vi "HEWH Emerson Data.vi"(7 "Status":T2, 8 "error in (no error)":errorcluster, 10 "Emerson Flow Meter Data Input":T1, 11 "name (unnamed)":string) -> (0 "error out":errorcluster, 3 "Emerson Flow Meter Data Output":T1)   [LabVIEW 2019]
uses:
  Utility/Type Definitions/UTILITY Notifier.ctl
  Drivers/Emerson 5700 Transmitter/Type Definitions/Emerson 5700 Data.ctl
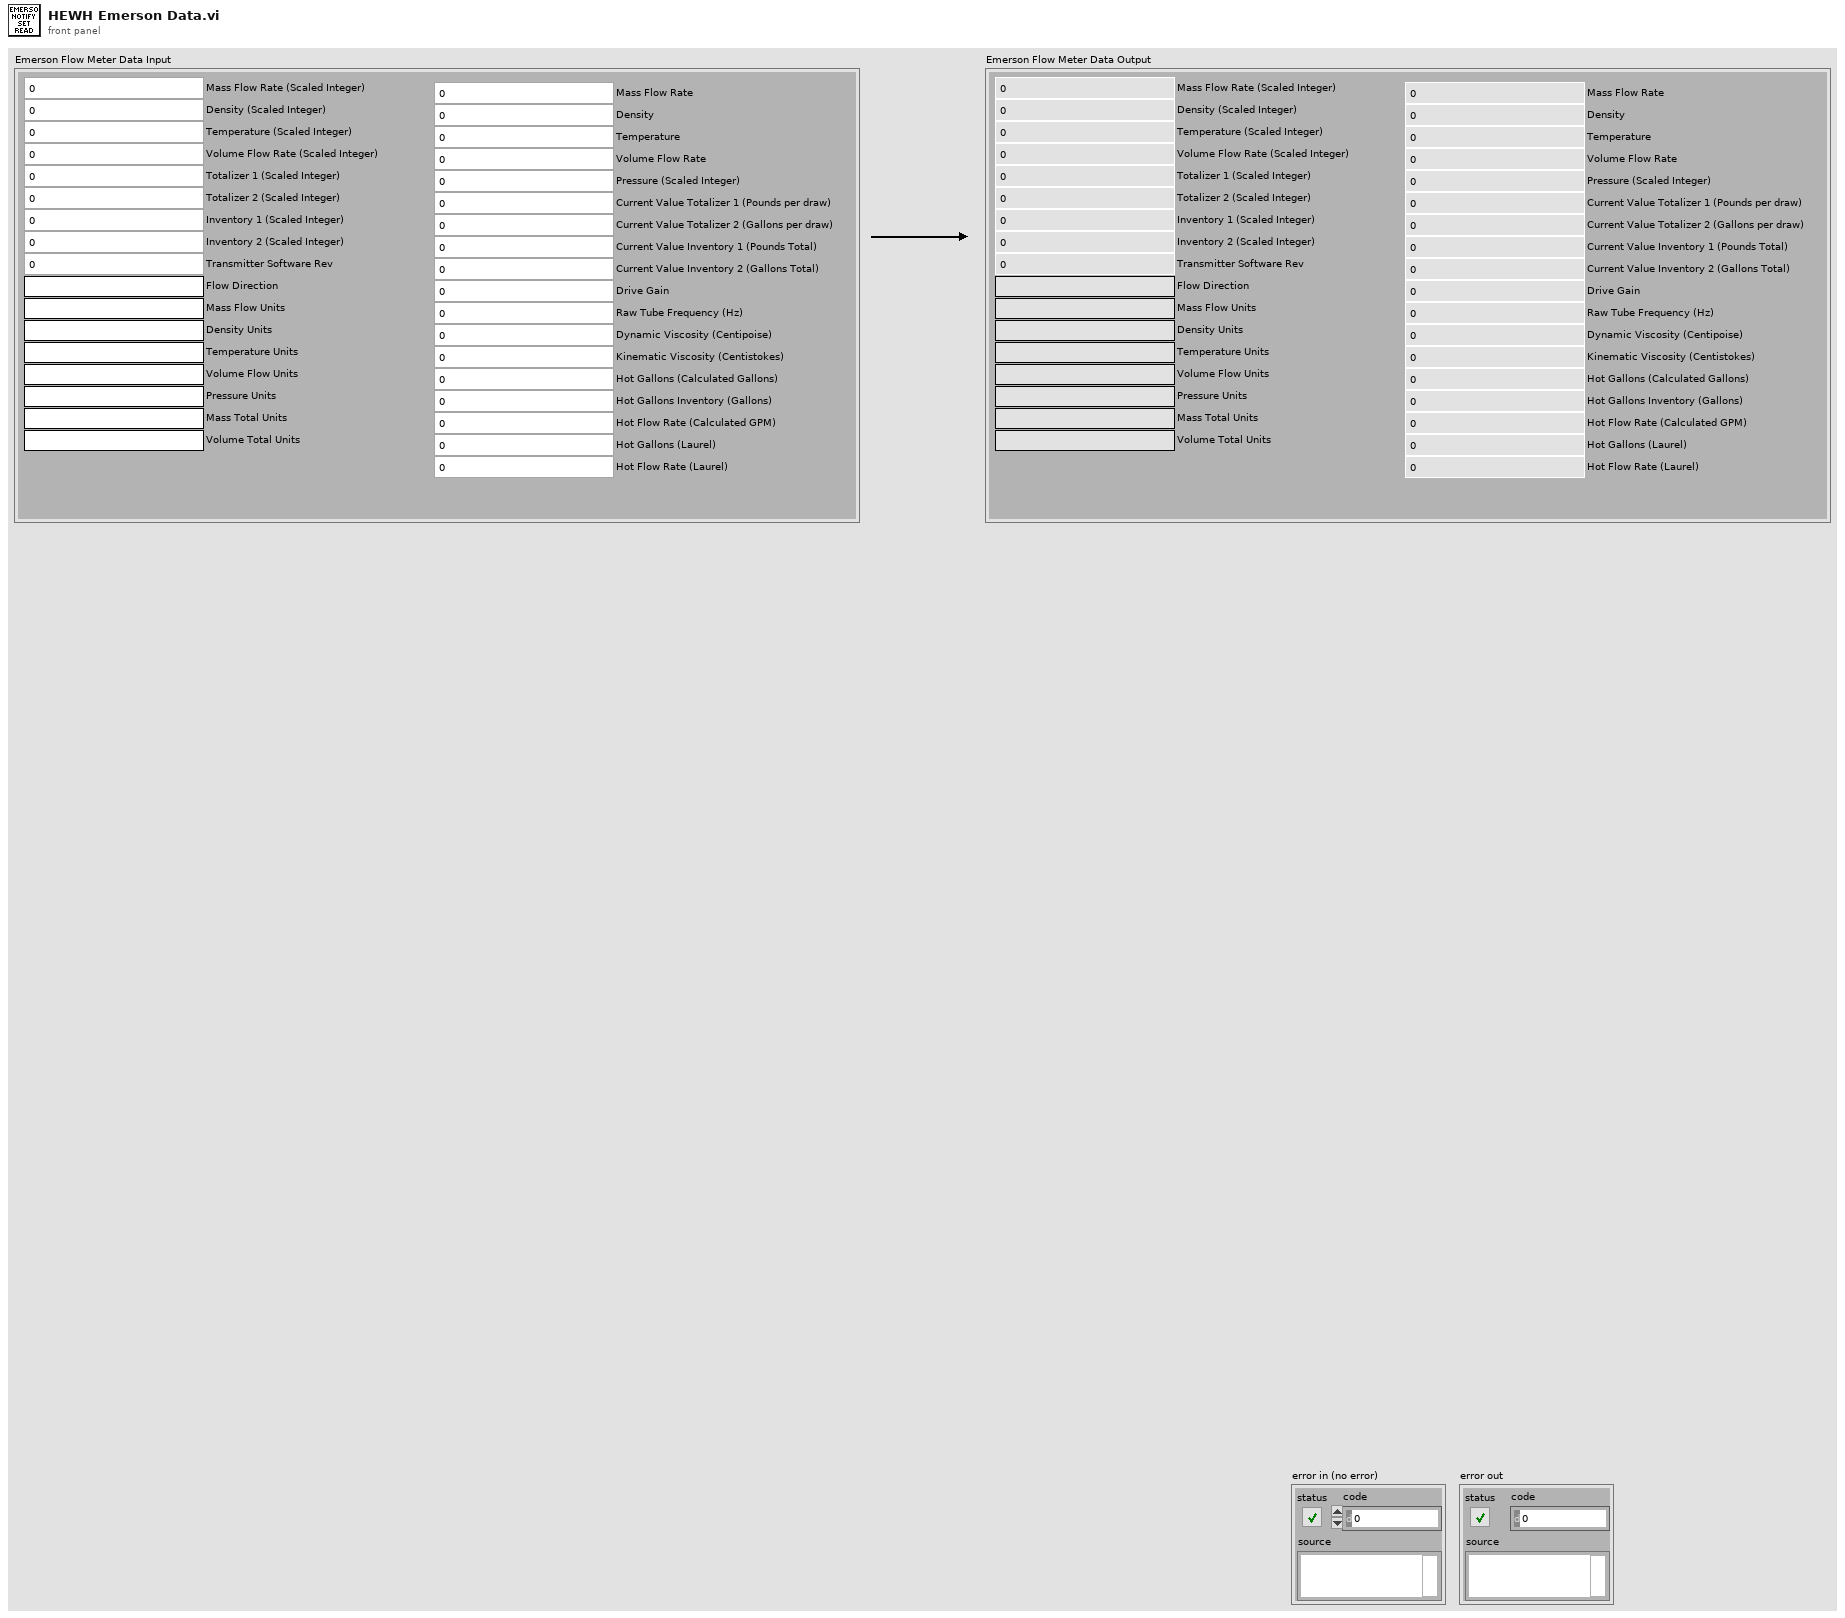
[diagram p1: front panel]
types:
  T1 = typedef "Emerson 5700 Data.ctl" = cluster{"Mass Flow Rate (Scaled Integer)":u16, "Density (Scaled Integer)":u16, "Temperature (Scaled Integer)":u16, "Volume Flow Rate (Scaled Integer)":u16, "Totalizer 1 (Scaled Integer)":u16, "Totalizer 2 (Scaled Integer)":u16, "Transmitter Software Rev":u16, "Flow Direction":string, "Mass Flow Units":string, "Density Units":string, "Temperature Units":string, "Volume Flow Units":string, "Pressure Units":string, "Mass Total Units":string, "Volume Total Units":string, "Inventory 1 (Scaled Integer)":u16, "Inventory 2 (Scaled Integer)":u16, "Mass Flow Rate":dbl, "Density":dbl, "Temperature":dbl, "Volume Flow Rate":dbl, "Pressure (Scaled Integer)":u16, "Current Value Totalizer 1 (Pounds per draw)":dbl, "Current Value Totalizer 2 (Gallons per draw)":dbl, "Current Value Inventory 1 (Pounds Total)":dbl, "Current Value Inventory 2 (Gallons Total)":dbl, "Drive Gain":dbl, "Raw Tube Frequency (Hz)":dbl, "Dynamic Viscosity (Centipoise)":dbl, "Kinematic Viscosity (Centistokes)":dbl, "Hot Gallons (Calculated Gallons)":dbl, "Hot Flow Rate (Calculated GPM)":dbl, "Hot Gallons Inventory (Gallons)":dbl, "Hot Flow Rate (Laurel)":dbl, "Hot Gallons (Laurel)":dbl}
  T2 = typedef "UTILITY Notifier.ctl" = enum16{"Set", "Read", "Release Ref"}
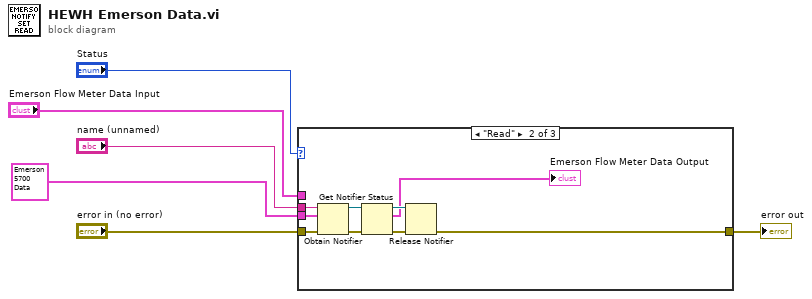
[diagram p0: block diagram]
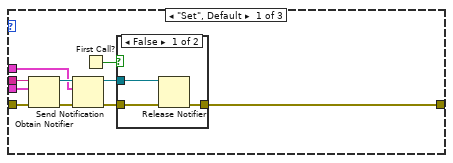
[diagram p2: hidden frame]
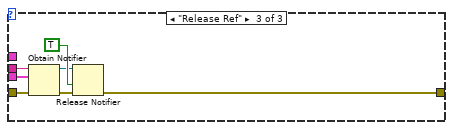
[diagram p4: hidden frame]
diagram:
  n1 = case shown="\"Read\"" "Status" {
    tunnel: [w7 w23 w32] -> w6
    tunnel: "error in (no error)" -> [w14 w27 w33]
    tunnel: "name (unnamed)" -> [w13 w26 w31]
    tunnel: T1 {"Mass Flow Rate (Scaled Integer)"=0, "Density (Scaled Integer)"=0, "Temperature (Scaled Integer)"=0, "Volume Flow Rate (Scaled Integer)"=0, "Totalizer 1 (Scaled Integer)"=0, "Totalizer 2 (Scaled Integer)"=0, "Transmitter Software Rev"=0, "Flow Direction"="", "Mass Flow Units"="", "Density Units"="", "Temperature Units"="", "Volume Flow Units"="", "Pressure Units"="", "Mass Total Units"="", "Volume Total Units"="", "Inventory 1 (Scaled Integer)"=0, "Inventory 2 (Scaled Integer)"=0, "Mass Flow Rate"=0.0, "Density"=0.0, "Temperature"=0.0, "Volume Flow Rate"=0.0, "Pressure (Scaled Integer)"=0, "Current Value Totalizer 1 (Pounds per draw)"=0.0, "Current Value Totalizer 2 (Gallons per draw)"=0.0, "Current Value Inventory 1 (Pounds Total)"=0.0, "Current Value Inventory 2 (Gallons Total)"=0.0, "Drive Gain"=0.0, "Raw Tube Frequency (Hz)"=0.0, "Dynamic Viscosity (Centipoise)"=0.0, "Kinematic Viscosity (Centistokes)"=0.0, "Hot Gallons (Calculated Gallons)"=0.0, "Hot Flow Rate (Calculated GPM)"=0.0, "Hot Gallons Inventory (Gallons)"=0.0, "Hot Flow Rate (Laurel)"=0.0, "Hot Gallons (Laurel)"=0.0} ("Emerson Flow Meter Data Input 2") -> [w11 w25 w30]
    tunnel: "Emerson Flow Meter Data Input" -> [w12 _ _]
    frame "Set", Default {
      n2 = Obtain Notifier(name (unnamed)=w13, notification data type=w11, error in (no error)=w14) -> (notifier out=w15:refnum<notifier>, error out=w16:errorcluster)  [unwired: 1 in, 1 out]
      n3 = Send Notification(notification=w12, notifier=w15, error in (no error)=w16) -> (notifier out=w9:refnum<notifier>, error out=w10:errorcluster)
      n4 = First Call?() -> (First Call?: T/F=w8:bool)
      n5 = case shown="False" w8 {
        tunnel: w10 -> [w19 w20]
        tunnel: [w18 w20] -> w7
        tunnel: w9 -> [w17 _]
        frame False {
          n6 = Release Notifier(notifier=w17, error in (no error)=w19) -> (error out=w18:errorcluster)  [unwired: 1 in, 2 out]
        }
        frame True {
        }
      }
    }
    frame "Read" {
      n7 = Obtain Notifier(name (unnamed)=w26, notification data type=w25, error in (no error)=w27) -> (notifier out=w28:refnum<notifier>, error out=w29:errorcluster)  [unwired: 1 in, 1 out]
      n8 = Get Notifier Status(notifier=w28, error in (no error)=w29) -> (notifier out=w22:refnum<notifier>, current notification=→"Emerson Flow Meter Data Output":T1, error out=w24:errorcluster)  [unwired: 2 out]
      n9 = Release Notifier(notifier=w22, error in (no error)=w24) -> (error out=w23:errorcluster)  [unwired: 1 in, 2 out]
    }
    frame "Release Ref" {
      n10 = Obtain Notifier(name (unnamed)=w31, notification data type=w30, error in (no error)=w33) -> (notifier out=w35:refnum<notifier>, error out=w34:errorcluster)  [unwired: 1 in, 1 out]
      n11 = Release Notifier(notifier=w35, force destroy? (F)=TRUE, error in (no error)=w34) -> (error out=w32:errorcluster)  [unwired: 2 out]
    }
  }
  "error out" <- w6
